vi "readWithDomain.vi"(6 "timeout (0)":i32, 8 "error in (no error)":errorcluster, 9 "bufferSize":i64, 11 "IStreamReader in":refnum<class "IStreamReader.lvclass">) -> (0 "error out":errorcluster, 1 "Reader Status out":refnum<class "IReaderStatus.lvclass">, 2 "Read Buffers":T1, 3 "IStreamReader out":refnum<class "IStreamReader.lvclass">)   [LabVIEW 2022 SP3, in "openDAQ.lvlib" / "IBaseObject.lvlib" / "IReader.lvlib" / "ISampleReader.lvlib" / "IStreamReader.lvlib" / "IStreamReader.lvclass"]
uses:
  <instrlib>/openDAQ/Public/Classes/IStreamReader/IStreamReader.lvclass
  C:/Program Files (x86)/National Instruments/LabVIEW 2022/instr.lib/openDAQ/Public/Classes/IBaseObject/IBaseObject.lvclass
  <instrlib>/openDAQ/Public/Classes/IReaderStatus/IReaderStatus.lvclass
  <instrlib>/openDAQ/Public/Classes/IMultiReaderStatus/IMultiReaderStatus.lvclass
  C:/Program Files (x86)/National Instruments/LabVIEW 2022/instr.lib/openDAQ/Public/Classes/IReaderStatus/IReaderStatus.lvclass
  <instrlib>/openDAQ/Public/Classes/IBaseObject/IBaseObject.lvclass/IBaseObject.ctl
  <instrlib>/openDAQ/Public/Classes/IBaseObject/Accessor/Read reference.vi
  <instrlib>/openDAQ/Public/Classes/IBaseObject/Accessor/Write reference.vi
  <instrlib>/openDAQ/Public/Classes/IStreamReader/IStreamReader.lvclass/IStreamReader.ctl
  <instrlib>/openDAQ/Binaries/Windows/x86/copendaq32.dll
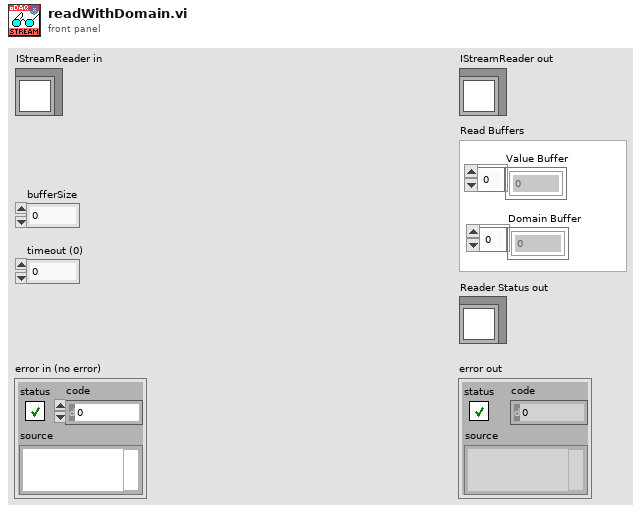
[diagram p1: front panel]
types:
  T1 = cluster{"Value Buffer":dbl[], "Domain Buffer":i64[]}
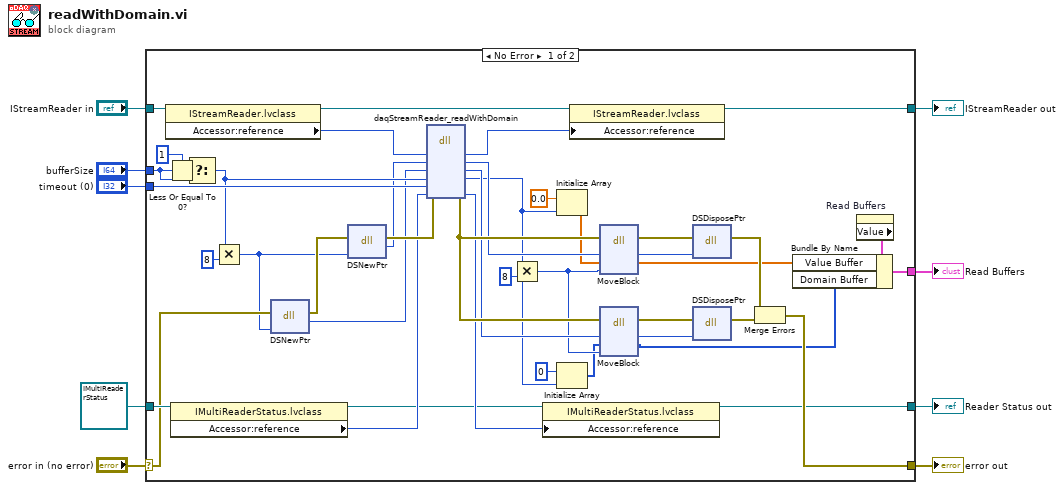
[diagram p0: block diagram]
diagram:
  n1 = case shown="No Error" "error in (no error)" {
    selector: "error in (no error)" -> [w25 w55]
    tunnel: [w50 w55] -> w8
    tunnel: [w45 w54] -> w6
    tunnel: "IStreamReader in" -> [w47 w54]
    tunnel: "bufferSize" -> [w34 _]
    tunnel: refnum<class "IMultiReaderStatus.lvclass"> refnum ("openDAQ.lvlib:IBaseObject.lvlib:IReaderStatus.lvlib:IMultiReaderStatus.lvlib:IMultiReaderStatus.lvclass") -> [w42 w53]
    tunnel: [w38 w53] -> w3
    tunnel: "timeout (0)" -> [w37 _]
    tunnel: [w13 _] -> w1
    frame No Error {
      n2 = property class="IStreamReader.lvclass"(reference=w47) -> (reference out=w46:refnum<class "IStreamReader.lvclass">, "Accessor:reference"=w44:i64)  [unwired: 1 in, 1 out]
      n3 = Less Or Equal To 0?(x=w34) -> (x <= 0?=w36:bool)
      n4 = property class="IMultiReaderStatus.lvclass"(reference=w42) -> (reference out=w39:refnum<class "IMultiReaderStatus.lvclass">, "Accessor:reference"=w41:i64)  [unwired: 1 in, 1 out]
      n5 = Select(t=i64 1, s=w36, f=w34) -> (s? t:f=w35:i64)
      n6 = Multiply(x=w35, y=i64 8) -> (x*y=w24:i64)
      n7 = dll-call lib="LabVIEW" fn="DSNewPtr"(error in=w25, "size"=w24) -> (error out=w49:errorcluster, "block*"=w23:i64)  [unwired: 3 in, 1 out]
      n8 = dll-call lib="LabVIEW" fn="DSNewPtr"(error in=w49, "size"=w24) -> (error out=w48:errorcluster, "block*"=w30:i64)  [unwired: 3 in, 1 out]
      n9 = dll-call lib="C:/Program Files (x86)/National Instruments/LabVIEW 2022/instr.lib/openDAQ/Binaries/Windows/x86/copendaq*.*" fn="daqStreamReader_readWithDomain"(error in=w48, "streamReader"=w44, "dataBuffers"=w30, "domain"=w23, "count"=w35, "timeout"=w37, "status"=w41) -> (error out=w52:errorcluster, "streamReader"=w43:i64, "dataBuffers"=w32:i64, "domain"=w22:i64, "count"=w11:i64, "status"=w40:i64)  [unwired: 4 in, 1 out]
      n10 = Multiply(x=w11, y=i64 8) -> (x*y=w20:i64)
      n11 = property class="IMultiReaderStatus.lvclass"(reference=w39, "Accessor:reference"=w40) -> (reference out=w38:refnum<class "IMultiReaderStatus.lvclass">)  [unwired: 1 in, 1 out]
      n12 = Initialize Array(0.0 ("element"), w11) -> (w21:dbl[])
      n13 = Initialize Array(i64 0 ("element"), w11) -> (w10:i64[])
      n14 = property class="IStreamReader.lvclass"(reference=w46, "Accessor:reference"=w43) -> (reference out=w45:refnum<class "IStreamReader.lvclass">)  [unwired: 1 in, 1 out]
      n15 = dll-call lib="LabVIEW" fn="MoveBlock"(error in=w52, "start"=w32, "destination"=w21, "size"=w20) -> (error out=w27:errorcluster, "start"=w26:i64, "destination"=w15:dbl[])  [unwired: 4 in, 1 out]
      n16 = dll-call lib="LabVIEW" fn="MoveBlock"(error in=w52, "start"=w22, "destination"=w10, "size"=w20) -> (error out=w19:errorcluster, "start"=w18:i64, "destination"=w14:i64[])  [unwired: 4 in, 1 out]
      n17 = dll-call lib="LabVIEW" fn="DSDisposePtr"(error in=w27, "pointer"=w26) -> (error out=w51:errorcluster)  [unwired: 4 in, 1 out]
      n18 = dll-call lib="LabVIEW" fn="DSDisposePtr"(error in=w19, "pointer"=w18) -> (error out=w17:errorcluster)  [unwired: 4 in, 1 out]
      n19 = Merge Errors(w51, w17) -> (w50:errorcluster)
      n20 = property on="Read Buffers" class="Clust (strict)"() -> ("Value"=w16:T1)  [unwired: 2 in, 2 out]
      n21 = Bundle By Name(cluster=w16, "Value Buffer"=w15, "Domain Buffer"=w14) -> (w13:T1)
    }
    frame Error {
    }
  }
  "error out" <- w8
  "IStreamReader out" <- w6
  "Reader Status out" <- w3
  "Read Buffers" <- w1
